vi "ConfigInstr.vi"(6 "InstrumentName":string, 7 "VisaRessIn":refnum<visa-resource-name>, 8 "error in (no error)":errorcluster caption="entrée d'erreur (pas d'erreur)", 9 "FirstClassInst":bool, 10 "Function":string, 11 "GenData In":refnum<class "PhotoLum.lvclass"> caption="DNL_LabVIEW Object in") -> (0 "error out":errorcluster caption="sortie d'erreur", 3 "GenData Out":refnum<class "PhotoLum.lvclass"> caption="DNL_LabVIEW Object out")   [LabVIEW 2019, in "PhotoLum.lvclass"]
uses:
  PhotoLum.lvclass
  C:/Programmes Labview/LabScanV1A/DevicesClass/BaseDevice/BaseDevice.lvclass
  PhotoLum_Func.ctl
  PhotoLum.lvclass/PhotoLum.ctl
  BaseDevice/BaseDevice.lvclass/BaseDevice.ctl
  BaseDevice/Accessor/SetShowInstrNm.vi
panel:
  in  "PhotoLum_Func":T1
  out "VisaRessOut":refnum<visa-resource-name>
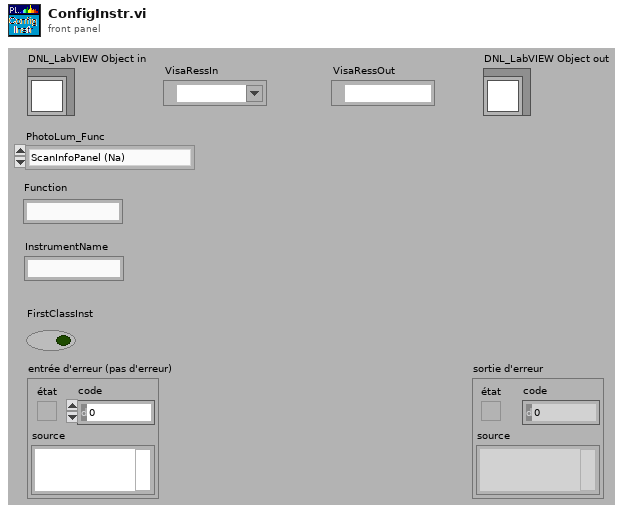
[diagram p1: front panel]
types:
  T1 = typedef "PhotoLum.lvclass/PhotoLum_Func.ctl" = enum16{"ScanInfoPanel (Na)", "MicroPLInfoPanel (NA)", "ExcimerInfoPan (NA)"}
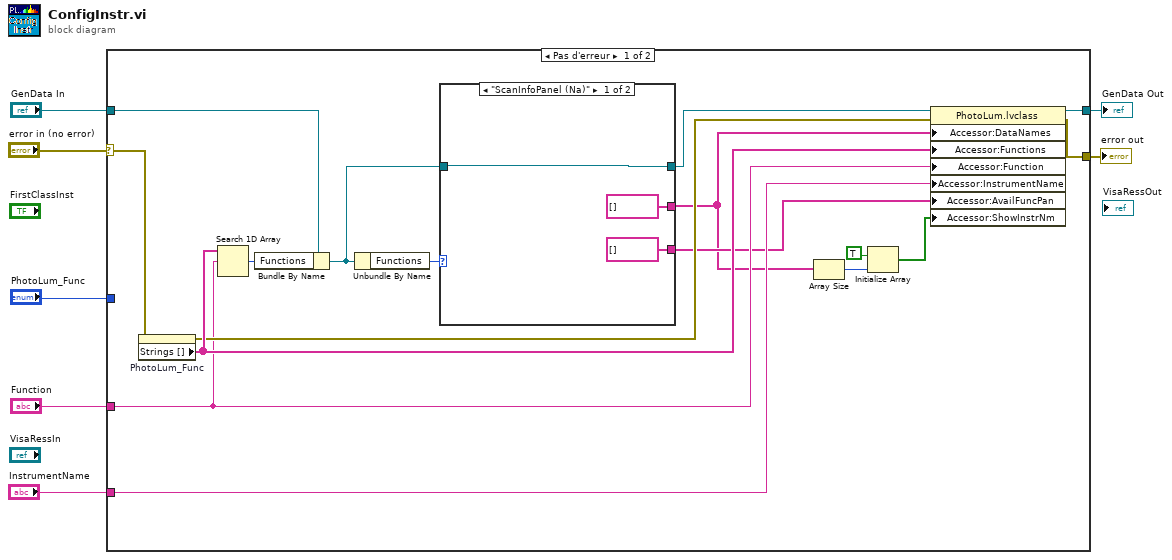
[diagram p0: block diagram]
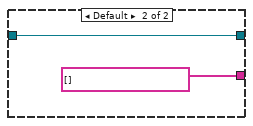
[diagram p2: hidden frame]
diagram:
  n1 = case shown="Pas d'erreur" "error in (no error)" {
    selector: "error in (no error)" -> [w18 w31]
    tunnel: [w24 w31] -> w6
    tunnel: "GenData In" -> [w19 w30]
    tunnel: [w23 w30] -> w4
    tunnel: "PhotoLum_Func" -> [_ _]
    tunnel: "Function" -> [w14 _]
    tunnel: "InstrumentName" -> [w13 _]
    frame No Error {
      n2 = property on="PhotoLum_Func" class="Énum (strict)"(error in=w18) -> (error out=w17:errorcluster, "Strings []"=w21:string[])  [unwired: 1 in, 1 out]
      n3 = Search 1D Array(1D array=w21, element=w14) -> (index of element=w20:i32)  [unwired: 1 in]
      n4 = Bundle By Name(cluster=w19, "Functions"=w20) -> (w16:refnum<class "PhotoLum.lvclass">)
      n5 = Unbundle By Name(w16) -> ("Functions"=w22:T1)
      n6 = case shown="\"ScanInfoPanel (Na)\"" w22 {
        tunnel: [string[] [] string[] []] -> w9
        tunnel: w16 -> [w27 w28]
        tunnel: [w27 w28] -> w15
        tunnel: [string[] [] _] -> w12
        frame "ScanInfoPanel (Na)" {
        }
        frame Default {
        }
      }
      n7 = Array Size(array=w9) -> (size(s)=w11:i32)
      n8 = Initialize Array(TRUE, w11) -> (w8:bool[])
      n9 = property class="PhotoLum.lvclass"(reference=w15, error in=w17, "Accessor:DataNames"=w9, "Accessor:Functions"=w21, "Accessor:Function"=w14, "Accessor:InstrumentName"=w13, "Accessor:AvailFuncPan"=w12, "Accessor:ShowInstrNm"=w8) -> (reference out=w23:refnum<class "PhotoLum.lvclass">, error out=w24:errorcluster)
    }
    frame Error {
    }
  }
  "error out" <- w6
  "GenData Out" <- w4
